vi "attributes-dependencies-test.vi"(8 "error in (no error)":errorcluster) -> (0 "error out":errorcluster)   [LabVIEW 2013]
uses:
  src/SMO/SMO.lvclass
  src/Support/Attribute/Attribute.lvclass/Attribute.ctl
  <vilib>/Utility/LVClass/Get LV Class Name.vi
  <vilib>/addons/_JKI Toolkits/Caraya/classes/Test/Test.lvclass
  <vilib>/addons/_JKI Toolkits/Caraya/classes/Assert/Assert.lvclass
  src/Support/Attribute/Attribute.lvclass
  src/Support/Attribute.Dependencies/Attribute.Dependencies.lvclass
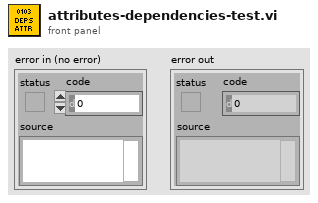
[diagram p1: front panel]
types:
  T1 = typedef "Attribute.Dependencies.lvclass/DependencyAttr--Cluster.ctl" = cluster{"Name":string, "GUID":string, "owned":bool, "shared":bool, "Level":string, "SMO":refnum<class "SMO.lvclass">}
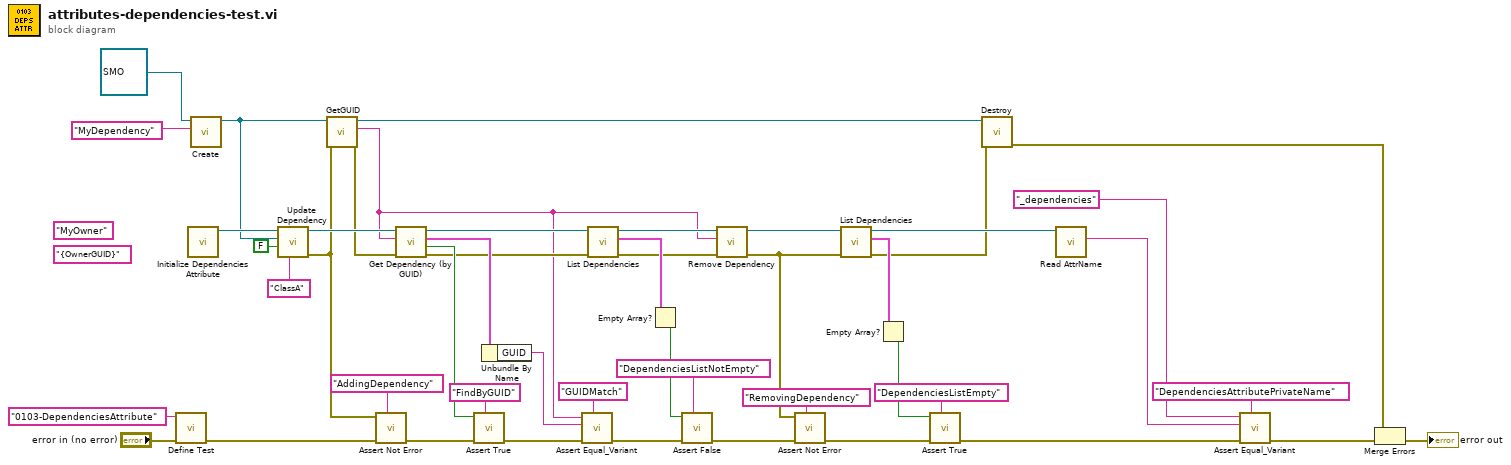
[diagram p0: block diagram]
diagram:
  (unwired) "{OwnerGUID}" ("Name")
  (unwired) "MyOwner" ("Name")
  n1 = call <vilib>:"Define Test.vi"("error in (no error)"="error in (no error)", "Label (VI Title)"="0103-DependenciesAttribute") -> ("error out"=w15:errorcluster)  [unwired: 9 in]
  n2 = call "Initialize Dependencies Attribute.vi"() -> ("Attribute.Dependencies"=w39:refnum<class "Attribute.Dependencies.lvclass">)  [unwired: 11 in]
  n3 = call "Create.vi"("Subsystem Name (optional)"="MyDependency" ("Name"), "SMO"=refnum<class "SMO.lvclass"> refnum) -> ("SMO out"=w35:refnum<class "SMO.lvclass">)  [unwired: 7 in, 2 out]
  n4 = call "Update Dependency.vi"("Level"="ClassA" ("Name"), "owned"=FALSE, "SMO"=w35, "Attribute.Dependencies in"=w39) -> ("error out"=w13:errorcluster, "Attribute.Dependencies out"=w34:refnum<class "Attribute.Dependencies.lvclass">)  [unwired: 6 in]
  n5 = call "GetGUID.vi"("error in (no error)"=w13, "SMO"=w35) -> ("error out"=w28:errorcluster, "GUID"=w22:string, "SMO out"=w6:refnum<class "SMO.lvclass">)  [unwired: 7 in]
  n6 = call <vilib>:"Assert Not Error.vi"("Label"="AddingDependency" ("Label (VI Title)"), "error in (no error)"=w15, "Not Error?"=w13) -> ("error out"=w14:errorcluster)  [unwired: 8 in]
  n7 = call "Get Dependency (by GUID).vi"("error in (no error)"=w28, "GUID"=w22, "Attribute.Dependencies in"=w34) -> ("error out"=w27:errorcluster, "found"=w33:bool, "Dependency"=w32:T1, "Attribute.Dependencies out"=w29:refnum<class "Attribute.Dependencies.lvclass">)  [unwired: 5 in]
  n8 = call <vilib>:"Assert True.vi"("Label"="FindByGUID" ("Label (VI Title)"), "error in (no error)"=w14, "True?"=w33) -> ("error out"=w31:errorcluster)  [unwired: 8 in]
  n9 = Unbundle By Name(w32) -> ("GUID"=w30:string)
  n10 = call <vilib>:"Assert Equal_Variant.vi"("Label"="GUIDMatch" ("Label (VI Title)"), "error in (no error)"=w31, "Y"=w30, "X"=w22) -> ("error out"=w26:errorcluster)  [unwired: 7 in]
  n11 = call "List Dependencies.vi"("error in (no error)"=w27, "Attribute.Dependencies in"=w29) -> ("error out"=w21:errorcluster, "Dependencies"=w25:T1[], "Attribute.Dependencies out"=w23:refnum<class "Attribute.Dependencies.lvclass">)  [unwired: 7 in]
  n12 = Empty Array?(array=w25) -> (empty?=w24:bool)
  n13 = call <vilib>:"Assert False.vi"("Label"="DependenciesListNotEmpty" ("Label (VI Title)"), "error in (no error)"=w26, "False?"=w24) -> ("error out"=w18:errorcluster)  [unwired: 8 in]
  n14 = call "Remove Dependency.vi"("error in (no error)"=w21, "GUID"=w22, "Attribute.Dependencies in"=w23) -> ("error out"=w19:errorcluster, "Attribute.Dependencies out"=w20:refnum<class "Attribute.Dependencies.lvclass">)  [unwired: 7 in]
  n15 = call <vilib>:"Assert Not Error.vi"("Label"="RemovingDependency" ("Label (VI Title)"), "error in (no error)"=w18, "Not Error?"=w19) -> ("error out"=w9:errorcluster)  [unwired: 8 in]
  n16 = call "List Dependencies.vi"("error in (no error)"=w19, "Attribute.Dependencies in"=w20) -> ("error out"=w5:errorcluster, "Dependencies"=w11:T1[], "Attribute.Dependencies out"=w7:refnum<class "Attribute.Dependencies.lvclass">)  [unwired: 7 in]
  n17 = Empty Array?(array=w11) -> (empty?=w10:bool)
  n18 = call <vilib>:"Assert True.vi"("Label"="DependenciesListEmpty" ("Label (VI Title)"), "error in (no error)"=w9, "True?"=w10) -> ("error out"=w8:errorcluster)  [unwired: 8 in]
  n19 = call "Destroy.vi"("error in (no error)"=w5, "SMO"=w6) -> ("error out"=w2:errorcluster)  [unwired: 9 in]
  n20 = call "Read AttrName.vi"("Attribute in"=w7) -> ("Attribute Name"=w42:string)  [unwired: 9 in, 1 out]
  n21 = call <vilib>:"Assert Equal_Variant.vi"("Label"="DependenciesAttributePrivateName" ("Label (VI Title)"), "error in (no error)"=w8, "Y"=w42, "X"="_dependencies" ("Label (VI Title)")) -> ("error out"=w4:errorcluster)  [unwired: 7 in]
  n22 = Merge Errors(w2, w4) -> (→"error out":errorcluster)
